vi "getRange.vi"(8 "error in (no error)":errorcluster, 10 "config":string, 11 "K2602FileReader in":refnum<class "K2602FileReader.lvclass">) -> (0 "error out":errorcluster, 2 "range":cluster{"current":dbl, "voltage":dbl}[](array[cluster]), 3 "K2602FileReader out":refnum<class "K2602FileReader.lvclass">)   [LabVIEW 2011, in "Tools.lvlib" / "Filing.lvlib" / "K2602FileReader.lvclass"]
uses:
  K2602FileReader.lvclass
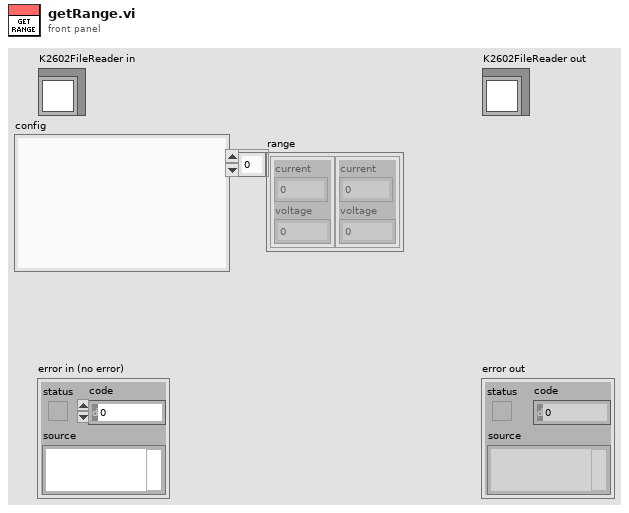
[diagram p1: front panel]
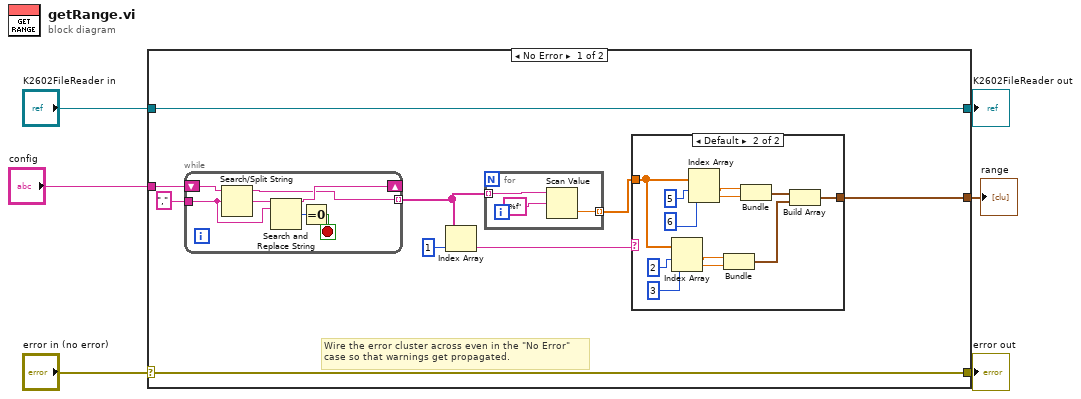
[diagram p0: block diagram]
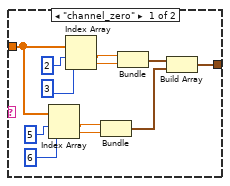
[diagram p2: hidden frame]
diagram:
  n1 = case shown="No Error" "error in (no error)" {
    selector: "error in (no error)" -> [w14 w51]
    tunnel: [w14 w51] -> w5
    tunnel: [w15 w50] -> w3
    tunnel: "K2602FileReader in" -> [w15 w50]
    tunnel: "config" -> [w10 _]
    tunnel: [w7 _] -> w1
    frame No Error {
      # "Wire the error cluster across even in the \"No Error\"\ncase so that warnings get propagated."
      n2 = while {
        tunnel: "," ("search string/char (-)") -> [w23]
        shift-right: [w20] -> _
        shift-left: w10 -> [w25]
        tunnel: [w19] -> w9 mode=indexing
        stop <- w21 stop-if-true
        n3 = Search/Split String(string=w25, search string/char (-)=w23) -> (substring before match=w19:string, match + rest of string=w24:string)  [unwired: 1 in, 1 out]
        n4 = Search and Replace String(input string=w24, search string=w23) -> (result string=w20:string, number of replacements=w22:i32)  [unwired: 6 in, 2 out]
        n5 = Equal To 0?(x=w22) -> (x = 0?=w21:bool)
      }
      n6 = Index Array(array=w9, index=1) -> (element=w12:string)
      n7 = for {
        tunnel: w9 -> [w18] mode=indexing
        tunnel: [w16] -> w8 mode=indexing
        n8 = Scan Value(string=w18, format string="%f") -> (value=w16:dbl)  [unwired: 1 in, 1 out]
      }
      n9 = case shown="Default" w12 {
        tunnel: w8 -> [w30 w42]
        tunnel: [w27 w39] -> w7
        frame "channel_zero" {
          n10 = Index Array(array=w30, index #1=5, index #2=6 ("index")) -> (element #1=w32:dbl, element #2=w31:dbl)
          n11 = Index Array(array=w30, index #1=2, index #2=3 ("index")) -> (element #1=w35:dbl, element #2=w34:dbl)
          n12 = Bundle(w32, w31) -> (w28:cluster{dbl, dbl})  [unwired: 1 in]
          n13 = Bundle(w35, w34) -> (w29:cluster{dbl, dbl})  [unwired: 1 in]
          n14 = Build Array(w29, w28) -> (w27:cluster{dbl, dbl}[])
        }
        frame Default {
          n15 = Index Array(array=w42, index #1=2, index #2=3 ("index")) -> (element #1=w44:dbl, element #2=w43:dbl)
          n16 = Index Array(array=w42, index #1=5, index #2=6 ("index")) -> (element #1=w47:dbl, element #2=w46:dbl)
          n17 = Bundle(w44, w43) -> (w40:cluster{dbl, dbl})  [unwired: 1 in]
          n18 = Bundle(w47, w46) -> (w41:cluster{dbl, dbl})  [unwired: 1 in]
          n19 = Build Array(w41, w40) -> (w39:cluster{dbl, dbl}[])
        }
      }
    }
    frame Error {
    }
  }
  "error out" <- w5
  "K2602FileReader out" <- w3
  "range" <- w1
